vi "Tosca-Open Visual Display.vi"(0 "Visual Display Settings":T1={"Use PTB"=TRUE, "IP Address"="localhost", "Port"=4926, "rect"={"left"=0, "top"=0, "width"=800, "height"=480}, "Full screen"=TRUE, "Open at start"=FALSE, "Monitor"=2, "Monitor size (in)"=8.0, "Monitor dist (in)"=24.0, "Photodiode Square"={"size"=50, "location"=enum."Bottom Left"}, "Background"=0.0}) -> (15 "error out":errorcluster)   [LabVIEW 2020]
uses:
  Tosca-Visual Display Settings.ctl
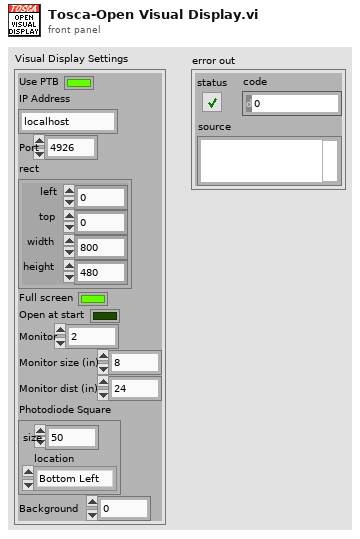
[diagram p1: front panel]
types:
  T1 = typedef "Tosca-Visual Display Settings.ctl" = cluster{"Use PTB":bool, "IP Address":string, "Port":i32, "rect":cluster{"left":i16, "top":i16, "width":i16, "height":i16}, "Full screen":bool, "Open at start":bool, "Monitor":i32, "Monitor size (in)":dbl, "Monitor dist (in)":dbl, "Photodiode Square":cluster{"size":i16, "location":enum16{"Bottom Left", "Top Left", "Top Right", "Bottom Right"}}, "Background":dbl}
  T2 = enum16{"Bottom Left", "Top Left", "Top Right", "Bottom Right"}
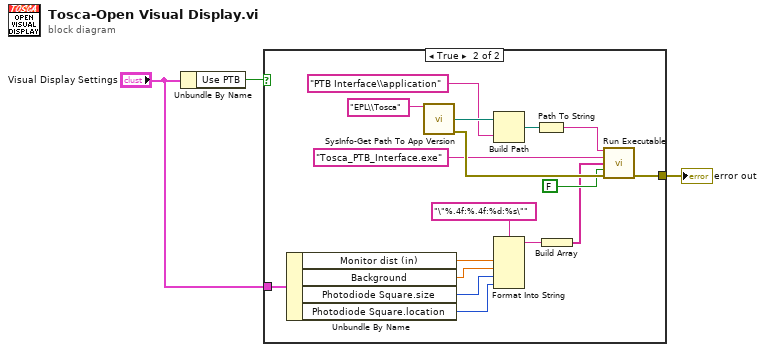
[diagram p0: block diagram]
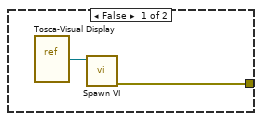
[diagram p2: hidden frame]
diagram:
  n1 = Unbundle By Name("Visual Display Settings") -> ("Use PTB"=w2:bool)
  n2 = case shown="True" w2 {
    tunnel: [w4 w14] -> w3
    tunnel: "Visual Display Settings" -> [_ w9]
    frame False {
      n3 = vi-ref "Tosca-Visual Display.vi"() -> (w5:refnum<vi>)
      n4 = call "Spawn VI.vi"("VI reference"=w5) -> ("error out"=w4:errorcluster)  [unwired: 9 in, 1 out]
    }
    frame True {
      n5 = Unbundle By Name(w9) -> ("Monitor dist (in)"=w12:dbl, "Background"=w11:dbl, "Photodiode Square.size"=w10:i16, "Photodiode Square.location"=w6:T2)
      n6 = call "SysInfo-Get Path To App Version.vi"("Path root"="EPL\\Tosca") -> ("Path without version"=w18:path, "error out"=w22:errorcluster)  [unwired: 12 in, 1 out]
      n7 = Build Path(base path=w18, name or relative path="PTB Interface\\application") -> (appended path=w17:path)
      n8 = Format Into String(format string="\"%.4f:%.4f:%d:%s\"" ("Command"), w12, w11, w10, w6) -> (resulting string=w8:string)  [unwired: 2 in, 1 out]
      n9 = Path To String(path=w17) -> (string=w16:string)
      n10 = Build Array(w8) -> (w7:string[])
      n11 = call "Run Executable.vi"("Folder"=w16, ".EXE name"="Tosca_PTB_Interface.exe", "args"=w7, "Wait (F)"=FALSE, "error in (no error)"=w22) -> ("error out"=w14:errorcluster)  [unwired: 10 in]
    }
  }
  "error out" <- w3
